vi "GainsSetting.vi"(3 "错误输入（无错误）":errorcluster, 4 "IMAQdx Session":T1, 5 "AnalogGainRaw":i64=227) -> (0 "错误输出":errorcluster, 2 "IMAQdx Session Out":T1)   [LabVIEW 2012]
uses:
  <vilib>/userDefined/High Color/IMAQdx.ctl
  <resource>/objmgr/imaqdx.rc
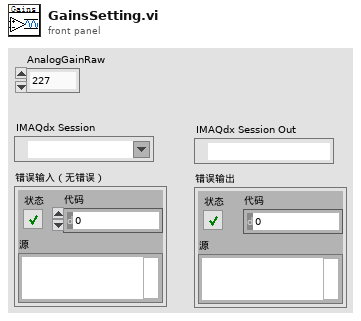
[diagram p1: front panel]
types:
  T1 = typedef "IMAQdx.ctl" = refnum<k21>
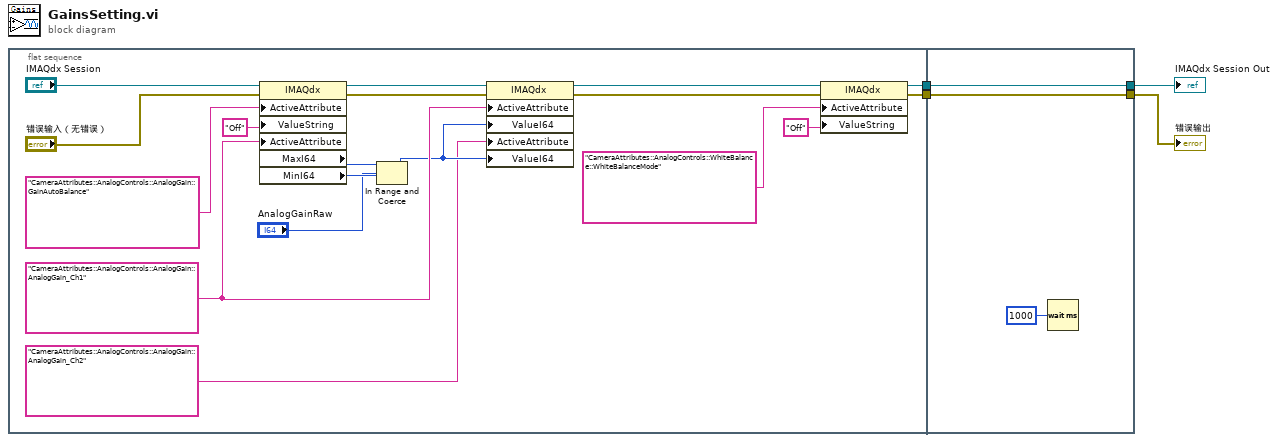
[diagram p0: block diagram]
diagram:
  n1 = flat-sequence {
    tunnel: [w16] -> w2
    tunnel: [w15] -> w1
    tunnel: [w24] -> w3
    tunnel: [w25] -> w4
    tunnel: w2 -> [w25]
    tunnel: w1 -> [w24]
    frame #0 {
      w10 = "CameraAttributes::AnalogControls::AnalogGain::AnalogGain_Ch1" ("ActiveAttribute")
      n2 = property class="IMAQdx"(reference="IMAQdx Session", error in="错误输入（无错误）", "ActiveAttribute"="CameraAttributes::AnalogControls::AnalogGain::GainAutoBalance", "ValueString"="Off", "ActiveAttribute"=w10) -> (reference out=w12:T1, error out=w11:errorcluster, "MaxI64"=w13:i64, "MinI64"=w14:i64)
      n3 = In Range and Coerce(upper limit=w13, x="AnalogGainRaw", lower limit=w14) -> (coerced(x)=w6:i64)  [unwired: 1 out]
      n4 = property class="IMAQdx"(reference=w12, error in=w11, "ActiveAttribute"=w10, "ValueI64"=w6, "ActiveAttribute"="CameraAttributes::AnalogControls::AnalogGain::AnalogGain_Ch2", "ValueI64"=w6) -> (reference out=w8:T1, error out=w7:errorcluster)
      n5 = property class="IMAQdx"(reference=w8, error in=w7, "ActiveAttribute"="CameraAttributes::AnalogControls::WhiteBalance::WhiteBalanceMode", "ValueString"="Off") -> (reference out=w16:T1, error out=w15:errorcluster)
    }
    frame #1 {
      n6 = Wait (ms)(milliseconds to wait=u32 1000 ("等待时间（毫秒）")) -> ()  [unwired: 1 out]
    }
  }
  "IMAQdx Session Out" <- w4
  "错误输出" <- w3
